vi "Handle Error.vi"(8 "error in (no error)":errorcluster, 11 "AF IMAQ Display in":refnum<class "HIJ Vision Display.lvclass">) -> (0 "error out":errorcluster, 2 "stop actor?":bool=TRUE, 3 "AF IMAQ Display out":refnum<class "HIJ Vision Display.lvclass">)   [LabVIEW 2014, in "HIJ Vision Display.lvlib" / "HIJ Vision Display.lvclass"]
doc: "(<B>Filename</B>: Actor Framework.lvlib:Actor.lvclass:Handle Error.vi)\n\nDefines how the actor handles an error that occurred while processing a message. By default, this method does nothing except stop the actor."
uses:
  HIJ Vision Display.lvclass
  Viewable Actor/ViewableActor/ViewableActor.lvclass
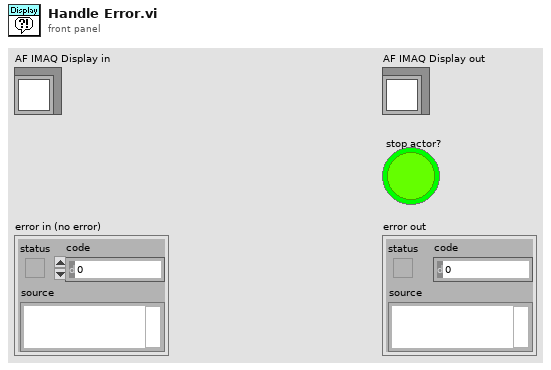
[diagram p1: front panel]
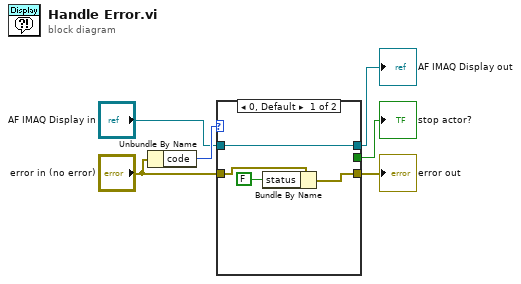
[diagram p0: block diagram]
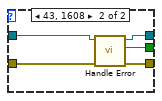
[diagram p2: hidden frame]
diagram:
  n1 = Unbundle By Name("error in (no error)") -> ("code"=w6:i32)
  n2 = case shown="0, Default" w6 {
    tunnel: [w9 w15] -> w2
    tunnel: [_ w14] -> w1
    tunnel: [w7 w13] -> w3
    tunnel: "error in (no error)" -> [w10 w12]
    tunnel: "AF IMAQ Display in" -> [w7 w11]
    frame 0, Default {
      n3 = Bundle By Name(cluster=w10, "status"=FALSE) -> (w9:errorcluster)
    }
    frame 43, 1608 {
      n4 = call-parent "Handle Error.vi"("error in (no error)"=w12, "Actor in"=w11) -> ("error out"=w15:errorcluster, "stop actor?"=w14:bool, "Actor out"=w13:refnum<class "HIJ Vision Display.lvclass">)  [unwired: 7 in]
    }
  }
  "AF IMAQ Display out" <- w3
  "error out" <- w2
  "stop actor?" <- w1
